vi "Motor_checkmotionisdone.vi"(0 "reference":refnum<k7>, 1 "error in (no error)":errorcluster) -> (2 "reference out":refnum<k7>, 3 "Motion is done":bool, 4 "error out":errorcluster)   [LabVIEW 2018]
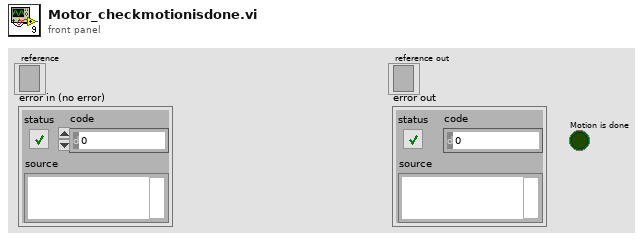
[diagram p1: front panel]
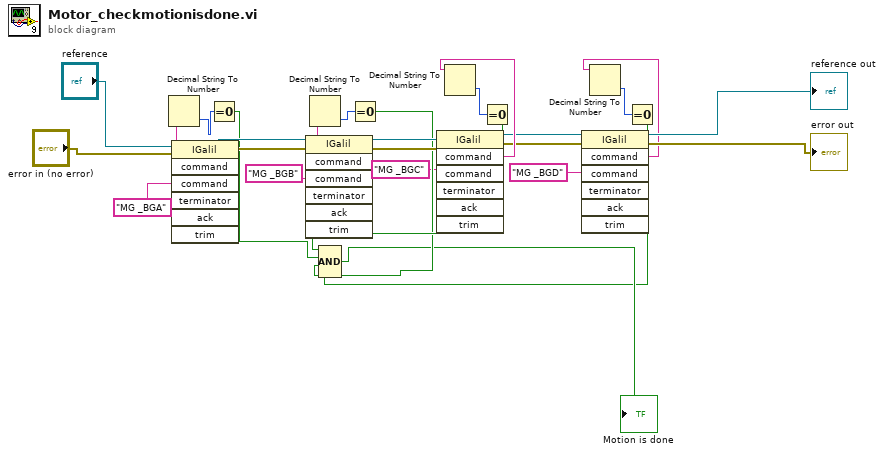
[diagram p0: block diagram]
diagram:
  n1 = invoke class="IGalil" method="command"(reference="reference", error in="error in (no error)", "command"="MG _BGA") -> (reference out=w22:refnum<k7>, error out=w21:errorcluster, "command"=w26:string)  [unwired: 4 in, 4 out]
  n2 = Decimal String To Number(string=w26) -> (number=w25:i32)  [unwired: 2 in, 1 out]
  n3 = Equal To 0?(x=w25) -> (x = 0?=w15:bool)
  n4 = invoke class="IGalil" method="command"(reference=w22, error in=w21, "command"="MG _BGB") -> (reference out=w19:refnum<k7>, error out=w18:errorcluster, "command"=w24:string)  [unwired: 4 in, 4 out]
  n5 = Decimal String To Number(string=w24) -> (number=w20:i32)  [unwired: 2 in, 1 out]
  n6 = Equal To 0?(x=w20) -> (x = 0?=w14:bool)
  n7 = invoke class="IGalil" method="command"(reference=w19, error in=w18, "command"="MG _BGC") -> (reference out=w7:refnum<k7>, error out=w6:errorcluster, "command"=w9:string)  [unwired: 4 in, 4 out]
  n8 = Decimal String To Number(string=w9) -> (number=w17:i32)  [unwired: 2 in, 1 out]
  n9 = Equal To 0?(x=w17) -> (x = 0?=w16:bool)
  n10 = invoke class="IGalil" method="command"(reference=w7, error in=w6, "command"="MG _BGD") -> (reference out=→"reference out":refnum<k7>, error out=→"error out":errorcluster, "command"=w1:string)  [unwired: 4 in, 4 out]
  n11 = Decimal String To Number(string=w1) -> (number=w8:i32)  [unwired: 2 in, 1 out]
  n12 = Equal To 0?(x=w8) -> (x = 0?=w3:bool)
  n13 = Compound Arithmetic op=AND(w16, w15, w14, w3) -> (→"Motion is done":bool)
